vi "Auton Scripting.vi"   [LabVIEW 2014]
uses:
  <vilib>/Rock Robotics/WPI/DriverStation/WPI_DriverStationRobotMode2.ctl
  Begin/Global Variables.vi
  <vilib>/Utility/file.llb/Write To Spreadsheet File (DBL).vi
types:
  T1 = typedef "WPI_DriverStationRobotMode2.ctl" = enum16{"Autonomous Disabled", "Autonomous Enabled", "Teleop Disabled", "Teleop Enabled", "Disconnected", "Finish", "Test Disabled", "Test Enabled", "Emergency Stopped"}
  T2 = cluster{"primitive":i32, "argument 1":dbl, "argument 2":dbl, "argument 3":dbl, "argument 4":dbl, "argument 5":dbl}
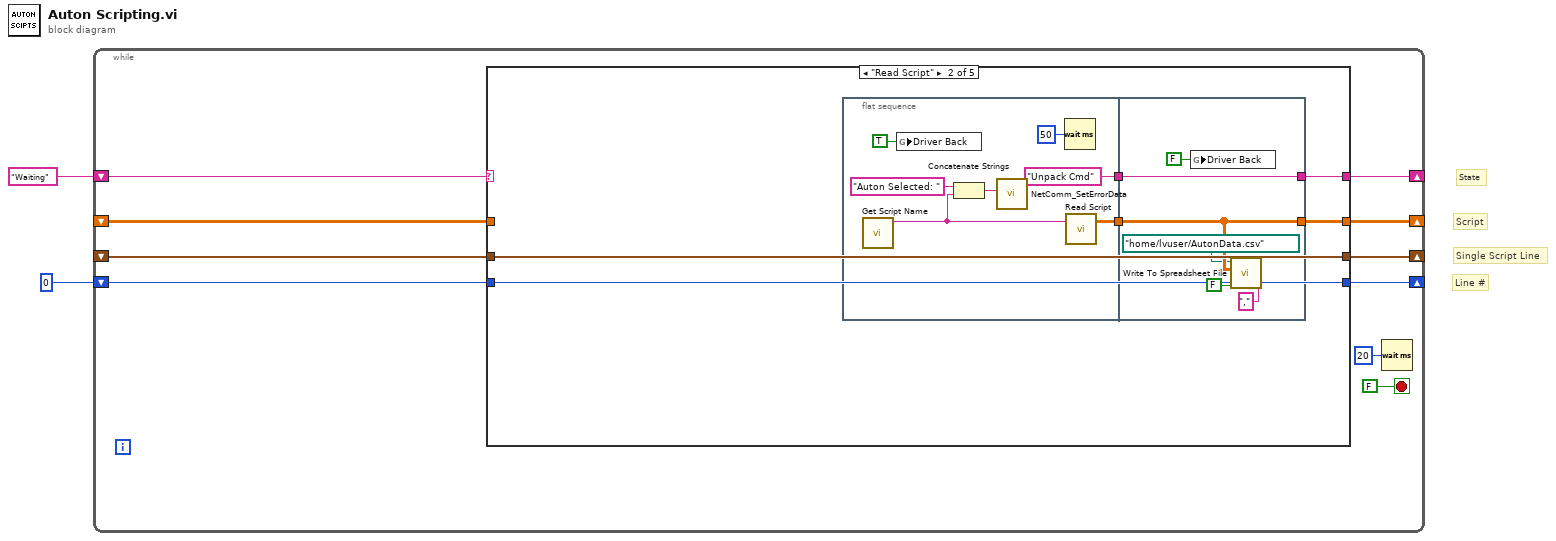
[diagram p0: block diagram]
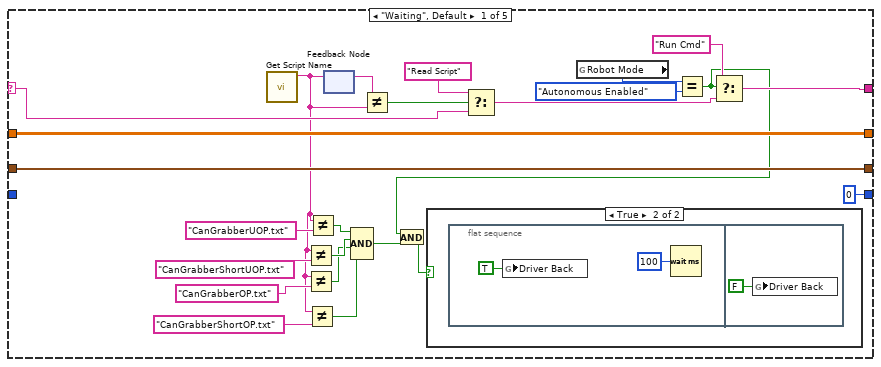
[diagram p2: hidden frame]
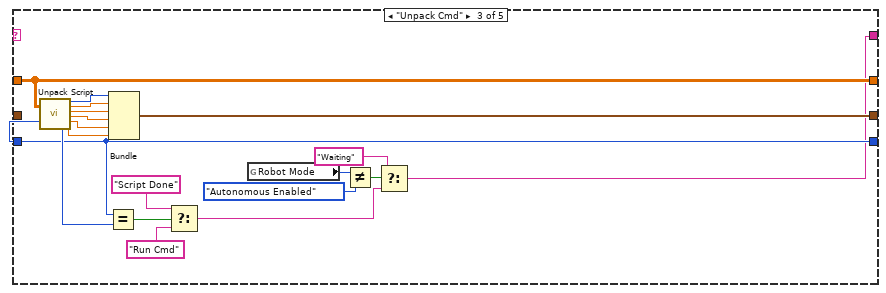
[diagram p4: hidden frame]
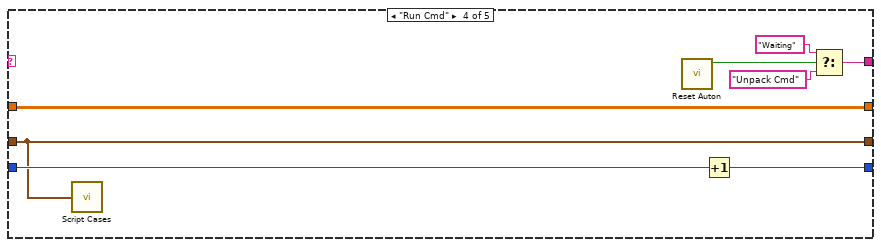
[diagram p5: hidden frame]
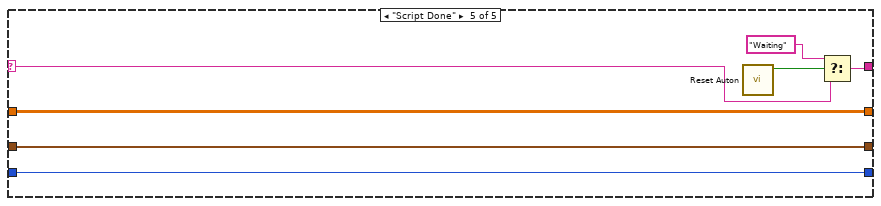
[diagram p6: hidden frame]
diagram:
  # "Line #"
  # "Single Script Line"
  # "Script"
  # "State"
  n1 = while {
    shift-right: [w10] -> _
    shift-left: "Waiting" ("Name") -> [w11]
    shift-right: [w9] -> _
    shift-left: _ -> [w8]
    shift-right: [w7] -> _
    shift-left: _ -> [w4]
    shift-right: [w5] -> _
    shift-left: u32 0 ("milliseconds to wait") -> [w6]
    stop <- FALSE stop-if-true
    n2 = case shown="\"Read Script\"" w11 {
      selector: w11 -> [w26 _ _ _ w89]
      tunnel: [w28 w44 w59 w83 w92] -> w10
      tunnel: [w33 w45 w70 w82 w88] -> w9
      tunnel: w8 -> [w33 _ w70 w82 w88]
      tunnel: [w27 w42 w71 w78 w87] -> w7
      tunnel: w6 -> [_ w43 w68 w80 w86]
      tunnel: [u32 0 ("milliseconds to wait") w43 w68 w79 w86] -> w5
      tunnel: w4 -> [w27 w42 _ w78 w87]
      frame "Waiting", Default {
        n3 = call "Get Script Name.vi"() -> ("Script Name"=w13:string)  [unwired: 11 in]
        n4 = Not Equal?(x=w13, y="CanGrabberShortUOP.txt") -> (x != y?=w18:bool)
        n5 = Not Equal?(x=w13, y="CanGrabberOP.txt") -> (x != y?=w16:bool)
        n6 = Not Equal?(x=w13, y="CanGrabberShortOP.txt") -> (x != y?=w14:bool)
        n7 = Not Equal?(x=w13, y="CanGrabberUOP.txt") -> (x != y?=w19:bool)
        n8 = feedback-in #1(w13) -> ()
        n9 = feedback #1() -> (w36:string)  [unwired: 1 in]
        n10 = Compound Arithmetic op=AND(w19, w18, w16, w14) -> (w20:bool)
        n11 = Not Equal?(x=w36, y=w13) -> (x != y?=w35:bool)
        n12 = Select(t="Read Script" ("Name"), s=w35, f=w26) -> (s? t:f=w32:string)
        n13 = global read "Global Variables.vi" "Robot Mode"() -> (w31:T1)
        n14 = Equal?(x=w31, y=WPI_DriverStationRobotMode2."Autonomous Enabled") -> (x = y?=w22:bool)
        n15 = And(x=w22, y=w20) -> (x .and. y?=w21:bool)
        n16 = case shown="True" w21 {
          frame False {
          }
          frame True {
            n17 = flat-sequence {
              frame #0 {
                n18 = global write "Global Variables.vi" "Driver Back"(TRUE ("Driver Back")) -> ()
                n19 = Wait (ms)(milliseconds to wait=u32 100) -> ()  [unwired: 1 out]
              }
              frame #1 {
                n20 = global write "Global Variables.vi" "Driver Back"(FALSE ("Driver Back")) -> ()
              }
            }
          }
        }
        n21 = Select(t="Run Cmd" ("Name"), s=w22, f=w32) -> (s? t:f=w28:string)
      }
      frame "Read Script" {
        n22 = flat-sequence {
          tunnel: [w52] -> w41
          tunnel: ["Unpack Cmd" ("Name")] -> w40
          tunnel: [w58] -> w44
          tunnel: [w56] -> w45
          tunnel: w41 -> [w56]
          tunnel: w40 -> [w58]
          frame #0 {
            n23 = call "Get Script Name.vi"() -> ("Script Name"=w49:string)  [unwired: 11 in]
            n24 = global write "Global Variables.vi" "Driver Back"(TRUE ("Driver Back")) -> ()
            n25 = Concatenate Strings("Auton Selected: " ("string"), w49) -> (w50:string)
            n26 = call <vilib>:"NetComm_SetErrorData.vi"("Error Data"=w50) -> ()  [unwired: 3 in, 8 out]
            n27 = Wait (ms)(milliseconds to wait=u32 50) -> ()  [unwired: 1 out]
            n28 = call "Read Script.vi"("script name"=w49) -> ("output array"=w52:dbl[][])  [unwired: 1 in, 1 out]
          }
          frame #1 {
            n29 = global write "Global Variables.vi" "Driver Back"(FALSE ("Driver Back")) -> ()
            n30 = call-poly <vilib>:"Write To Spreadsheet File.vi"("delimiter (\\t)"="," ("delimiter (\\t)"), "append to file? (new file:F)"=FALSE, "2D data"=w56, "file path (dialog if empty)"=path "/home/lvuser/AutonData.csv" ("file path (use dialog)")) -> ()  [unwired: 4 in, 1 out]
          }
        }
      }
      frame "Unpack Cmd" {
        n31 = call "Unpack Script.vi"("script"=w70, "index"=w68) -> ("# of primitives"=w69:i32, "primitive"=w77:i32, "argument 1"=w76:dbl, "argument 2"=w75:dbl, "argument 3"=w74:dbl, "argument 4"=w73:dbl, "argument 5"=w72:dbl)  [unwired: 11 in]
        n32 = Equal?(x=w68, y=w69) -> (x = y?=w67:bool)
        n33 = Bundle("primitive"=w77, "argument 1"=w76, "argument 2"=w75, "argument 3"=w74, "argument 4"=w73, "argument 5"=w72) -> (w71:T2)  [unwired: 1 in]
        n34 = Select(t="Script Done" ("Name"), s=w67, f="Run Cmd" ("Name")) -> (s? t:f=w61:string)
        n35 = global read "Global Variables.vi" "Robot Mode"() -> (w64:T1)
        n36 = Not Equal?(x=w64, y=WPI_DriverStationRobotMode2."Autonomous Enabled") -> (x != y?=w62:bool)
        n37 = Select(t="Waiting", s=w62, f=w61) -> (s? t:f=w59:string)
      }
      frame "Run Cmd" {
        n38 = call "Script Cases.vi"("Primitives & Arguments"=w78) -> ()
        n39 = call "Reset Auton.vi"() -> ("Reset Auton"=w81:bool)  [unwired: 11 in]
        n40 = Increment(x=w80) -> (x+1=w79:u32)
        n41 = Select(t="Waiting" ("Name"), s=w81, f="Unpack Cmd" ("Name")) -> (s? t:f=w83:string)
      }
      frame "Script Done" {
        n42 = call "Reset Auton.vi"() -> ("Reset Auton"=w91:bool)  [unwired: 11 in]
        n43 = Select(t="Waiting" ("Name"), s=w91, f=w89) -> (s? t:f=w92:string)
      }
    }
    n44 = Wait (ms)(milliseconds to wait=u32 20) -> ()  [unwired: 1 out]
  }
